vi "HISW_2_PAQ10sec.vi"(8 "error in (no error)":errorcluster, 10 "PAQdatagram IN":T3 {"data" format="%.2f"; "status" format="%08x"}, 11 "AVPP in":refnum<class "AVPP.lvclass">) -> (0 "error out":errorcluster, 2 "Next_Level":T1, 3 "AVPP out":refnum<class "AVPP.lvclass">)   [LabVIEW 2014]
doc: "Process the Saving of 10 seconds samples towards the FAMM"
uses:
  AVPP.lvclass
  HISW/controls/typedef_PAQdatagram.ctl
  FAMM/controls/typedef_AverageAction.ctl
  FAMM/controls/typedef_Level.ctl
  FAMM/controls/MemStoreDatagram.ctl
  FAMM/FAMM.lvclass
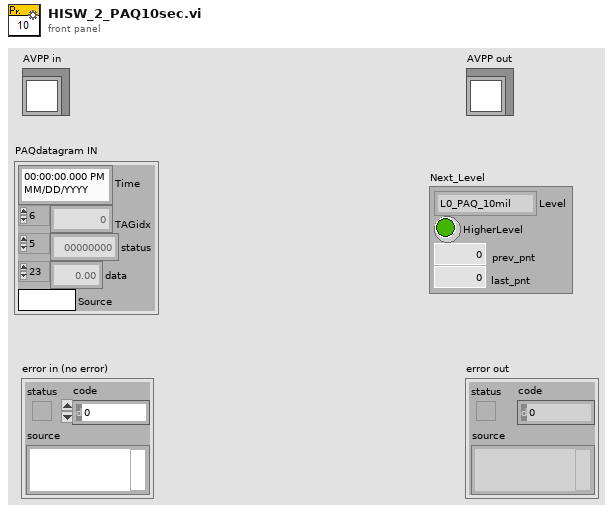
[diagram p1: front panel]
types:
  T1 = typedef "FAMM.lvclass/typedef_AverageAction.ctl" = cluster{"Level":T2, "HigherLevel":bool, "prev_pnt":i32, "last_pnt":i32}
  T2 = typedef "FAMM.lvclass/typedef_Level.ctl" = enum16{"L0_PAQ_10mil", "L0_PAQ_100mil", "L1_PAQ_100mil", "L2_PAQ_1sec", "L3_PAQ_10sec", "L4_PAQ_1min", "L5_PAQ_10min", "L6_PAQ_2hr", "L7_PAQ_1day", "L8_PAQ_1wk", "L1_PAQ_1sec", "L2_PAQ_10sec", "L3_PAQ_1min", "L4_PAQ_10min", "L5_PAQ_2hr", "L6_PAQ_1day", "L7_PAQ_1wk", "L0_PAQ_1sec", "L1_PAQ_10sec", "L2_PAQ_1min", "L3_PAQ_10min", "L4_PAQ_2hr", "L5_PAQ_1day", "L6_PAQ_1wk", "L0_PAQ_10sec", "L1_PAQ_1min", "L2_PAQ_10min", "L3_PAQ_2hr", "L4_PAQ_1day", "L5_PAQ_1wk"}
  T3 = typedef "typedef_PAQdatagram.ctl" = cluster{"Time":timestamp, "TAGidx":i32[], "status":u32[], "data":dbl[], "Source":string}
  T4 = typedef "FAMM.lvclass/MemStoreDatagram.ctl" = cluster{"Time":dbl, "TagIndex":i32[], "data":dbl[], "max":dbl[], "min":dbl[], "status":u32[], "Source":string}
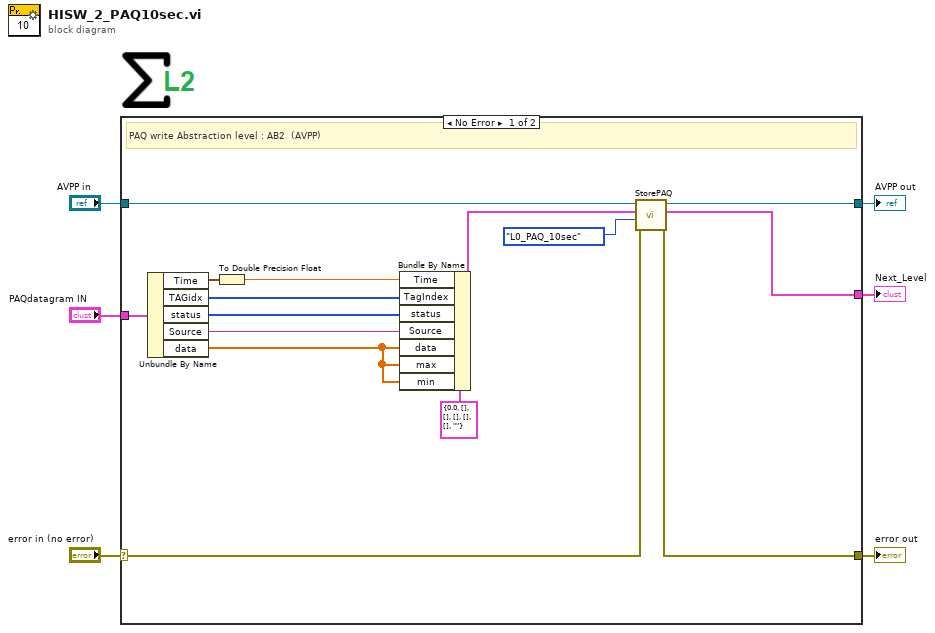
[diagram p0: block diagram]
diagram:
  n1 = case shown="No Error" "error in (no error)" {
    selector: "error in (no error)" -> [w10 w23]
    tunnel: [w9 w23] -> w5
    tunnel: [w21 w22] -> w3
    tunnel: "AVPP in" -> [w15 w22]
    tunnel: "PAQdatagram IN" -> [w19 _]
    tunnel: [w8 _] -> w1
    frame No Error {
      # "PAQ write Abstraction level : AB2  (AVPP)"
      n2 = Unbundle By Name(w19) -> ("Time"=w18:timestamp, "TAGidx"=w16:i32[], "status"=w14:u32[], "Source"=w13:string, "data"=w11:dbl[])
      n3 = To Double Precision Float(number=w18) -> (double precision float=w17:dbl)
      n4 = Bundle By Name(cluster=T4 {"Time"=0.0, "TagIndex"=[], "data"=[], "max"=[], "min"=[], "status"=[], "Source"=""} ("StoreDatagram"), "Time"=w17, "TagIndex"=w16, "status"=w14, "Source"=w13, "data"=w11, "max"=w11, "min"=w11) -> (w12:T4)
      n5 = call "StorePAQ.vi"("error in (no error)"=w10, "Level"=typedef_Level."L0_PAQ_10sec" ("Enum"), "StoreDatagram"=w12, "FAMM in"=w15) -> ("error out"=w9:errorcluster, "Next_Level"=w8:T1, "FAMM out"=w21:refnum<class "AVPP.lvclass">)  [unwired: 5 in]
    }
    frame Error {
    }
  }
  "error out" <- w5
  "AVPP out" <- w3
  "Next_Level" <- w1
